vi "Read File.vi"(7 "Channel Direction":string="Empty", 8 "error in (no error)":errorcluster, 11 "ConfigFile in":refnum<class "ConfigFile.lvclass">) -> (0 "error out":errorcluster, 2 "Channels":refnum<class "Channel.lvclass">[](array[class]), 3 "ConfigFile out":refnum<class "ConfigFile.lvclass">)   [LabVIEW 2020, in "ImportExport.lvlib"]
uses:
  ImportExport.lvlib
  ConfigFile/ConfigFile.lvclass
  built/windows/Channel.lvlibp/Channel.lvclass
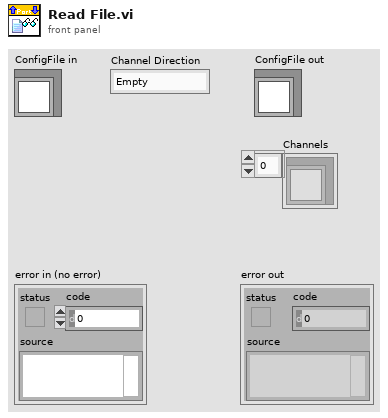
[diagram p1: front panel]
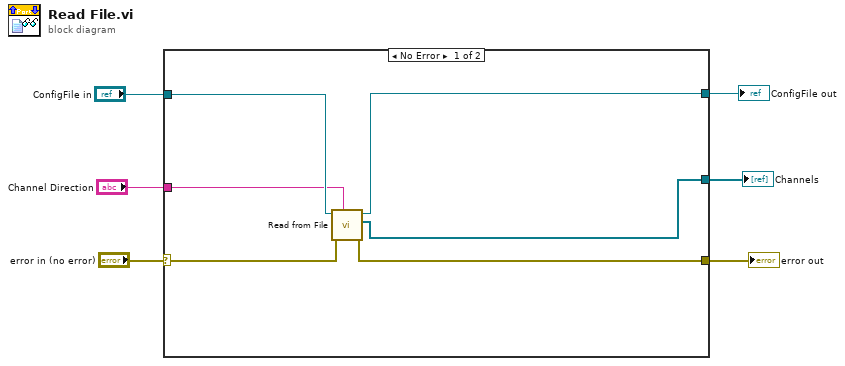
[diagram p0: block diagram]
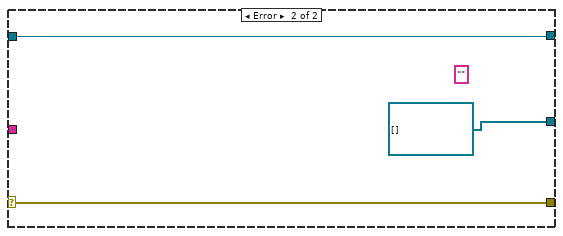
[diagram p2: hidden frame]
diagram:
  n1 = case shown="No Error" "error in (no error)" {
    selector: "error in (no error)" -> [w10 w15]
    tunnel: "ConfigFile in" -> [w12 w14]
    tunnel: [w8 w15] -> w5
    tunnel: [w11 w14] -> w4
    tunnel: [w7 refnum<class "Channel.lvclass">[] [] ("Channels")] -> w2
    tunnel: "Channel Direction" -> [w9 _]
    frame No Error {
      n2 = call-dynamic "Read from File.vi"("Channel Direction"=w9, "error in (no error)"=w10, "ConfigFile in"=w12) -> ("error out"=w8:errorcluster, "Channels"=w7:refnum<class "Channel.lvclass">[], "ConfigFile out"=w11:refnum<class "ConfigFile.lvclass">)  [unwired: 6 in]
    }
    frame Error {
      (unwired) "" ("Channel Direction")
    }
  }
  "error out" <- w5
  "ConfigFile out" <- w4
  "Channels" <- w2
